vi "배열 중복 제거 실습.vi"() -> ()   [LabVIEW 2020]
panel:
  out "배열 2":dbl[](array[numeric])
  out "배열":dbl[](array[numeric])
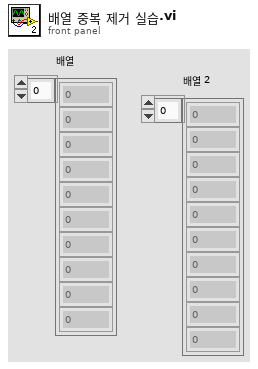
[diagram p1: front panel]
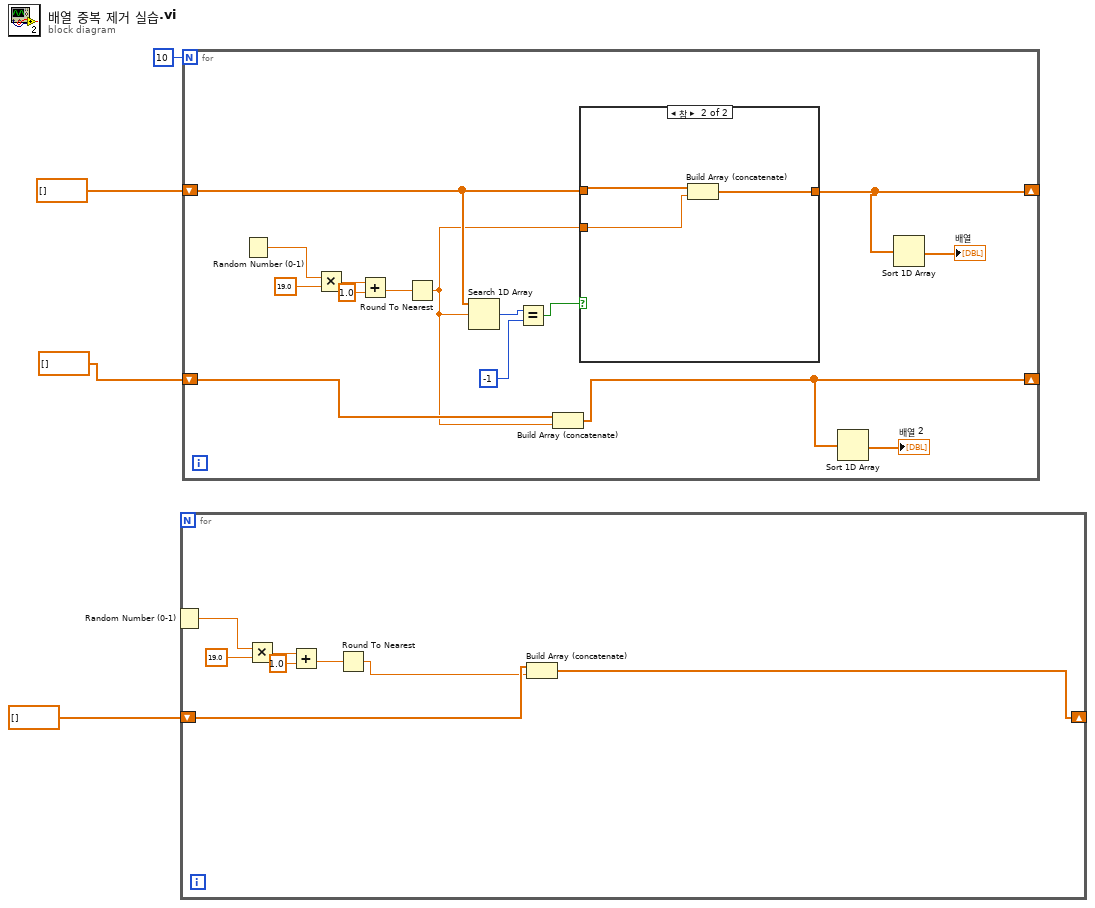
[diagram p0: block diagram]
diagram:
  n1 = for {
    shift-right: [w5] -> _
    shift-left: dbl[] [] -> [w7]
    n2 = Random Number (0-1)() -> (number: 0 to 1=w11:dbl)
    n3 = Multiply(x=w11, y=19.0) -> (x*y=w10:dbl)
    n4 = Add(x=w10, y=1.0) -> (x+y=w8:dbl)
    n5 = Round To Nearest(number=w8) -> (nearest integer value=w6:dbl)
    n6 = Build Array (concatenate)(w7, w6) -> (w5:dbl[])
  }
  n7 = for {
    N: 10 -> [_]
    shift-right: [w18] -> _
    shift-left: dbl[] [] -> [w23]
    shift-right: [w13] -> _
    shift-left: dbl[] [] -> [w16]
    n8 = Random Number (0-1)() -> (number: 0 to 1=w26:dbl)
    n9 = Multiply(x=w26, y=19.0) -> (x*y=w25:dbl)
    n10 = Add(x=w25, y=1.0) -> (x+y=w22:dbl)
    n11 = Round To Nearest(number=w22) -> (nearest integer value=w15:dbl)
    n12 = Search 1D Array(1D array=w23, element=w15) -> (index of element=w21:i32)  [unwired: 1 in]
    n13 = Equal?(x=w21, y=-1) -> (x = y?=w19:bool)
    n14 = Build Array (concatenate)(w16, w15) -> (w13:dbl[])
    n15 = case shown="참" w19 {
      tunnel: w23 -> [w28 w31]
      tunnel: w15 -> [_ w30]
      tunnel: [w28 w29] -> w18
      frame False {
      }
      frame True {
        n16 = Build Array (concatenate)(w31, w30) -> (w29:dbl[])
      }
    }
    n17 = Sort 1D Array(array=w13) -> (sorted array=→"배열 2":dbl[])
    n18 = Sort 1D Array(array=w18) -> (sorted array=→"배열":dbl[])
  }
